vi "BCU参数读取-Auto.vi"(8 "CAN端口":u16(ring), 9 "设备索引号":u16(ring), 10 "CAN卡类型":u32(ring)=21, 11 "Myindex":dbl=1.0) -> (3 "成功":bool)   [LabVIEW 2013] (continued)
                      w1344 = string[][] []
                      w1357 = "总信息" ("section")
                      n843 = local write "路径"(w1343) -> ()
                      n844 = call <vilib>:"Open Config Data.vi"("create file if necessary (T)"=FALSE, "configuration file path"=w1343) -> ("error out"=w1348:errorcluster, "refnum"=w1347:T25)  [unwired: 7 in, 1 out]
                      n845 = call <vilib>:"Get Key Names.vi"("section"=w1357, "error in (no error)"=w1348, "refnum"=w1347) -> ("key names"=w1356:string[], "refnum out"=w1358:T25)  [unwired: 5 in, 2 out]
                      n846 = for {
                        tunnel: w1358 -> [w1364]
                        tunnel: w1357 -> [w1363]
                        tunnel: w1356 -> [w1362] mode=indexing
                        tunnel: [w1361] -> w1353 mode=indexing
                        n847 = call-poly <vilib>:"Read Key.vi"("section"=w1363, "key"=w1362, "refnum"=w1364) -> ("value"=w1361:string)  [unwired: 5 in, 3 out]
                      }
                      n848 = Index Array(array=w1353) -> (element #1=w1346:string, element #2=w1351:string)  [unwired: 2 in]
                      n849 = Decimal String To Number(string=w1346) -> (number=w1345:i32)  [unwired: 2 in, 1 out]
                      n850 = Concatenate Strings("正在读取" ("字符串"), w1351, "的配置文件" ("字符串")) -> (w1349:string)
                      n851 = Build Array(w1349) -> (w1354:string[])
                      n852 = call "表格编辑.vi"("新元素/子数组"=w1354, "活动单元格:单元格背景色"=u32 6618880, "MCListbox引用句柄"=w1360) -> ()  [unwired: 9 out]
                      n853 = local write "项目信息"(w1344) -> ()
                      n854 = local write "项目信息 2"(w1344) -> ()
                    }
                    frame #1 {
                      w1535 = 20 ("长度")
                      w1576 = "主板" ("section")
                      n855 = call <vilib>:"Get Key Names.vi"("section"=w1576, "refnum"=w1575) -> ("key names"=w1377:string[], "refnum out"=w1577:T25)  [unwired: 6 in, 2 out]
                      n856 = for {
                        tunnel: w1577 -> [w1589]
                        tunnel: w1576 -> [w1588]
                        tunnel: w1377 -> [w1587] mode=indexing
                        tunnel: [w1586] -> w1376 mode=indexing
                        n857 = call-poly <vilib>:"Read Key.vi"("section"=w1588, "key"=w1587, "refnum"=w1589) -> ("value"=w1586:string)  [unwired: 5 in, 3 out]
                      }
                      n858 = Search 1D Array(1D array=w1377, element="总电压过高一级" ("元素"), start index (0)=0 ("开始索引(0)")) -> (index of element=w1457:i32)
                      n859 = Search 1D Array(1D array=w1377, element="风机开启温度" ("元素"), start index (0)=w1457) -> (index of element=w1448:i32)
                      n860 = Search 1D Array(1D array=w1377, element="电池串联" ("元素"), start index (0)=w1448) -> (index of element=w1446:i32)
                      n861 = Decrement(x=w1457) -> (x-1=w1574:i32)
                      n862 = Array Subset(array=w1377, index=1 ("索引"), length=w1574) -> (w1422:string[])
                      n863 = Array Subset(array=w1376, index=1 ("索引"), length=w1574) -> (w1419:string[])
                      n864 = Delete From Array(array=w1419, length=7 ("长度"), index=0 ("索引")) -> (deleted portion=w1416:string[], array with subset deleted=w1366:string[])
                      n865 = Delete From Array(array=w1422, length=7 ("长度"), index=0 ("索引")) -> (array with subset deleted=w1375:string[])  [unwired: 1 out]
                      n866 = Search 1D Array(1D array=w1377, element="分流器型号" ("元素")) -> (index of element=w1380:i32)  [unwired: 1 in]
                      n867 = Index Array(array=w1376, index=0 ("索引")) -> (element=w1550:string)
                      n868 = Decimal String To Number(string=w1550) -> (number=w1367:i32)  [unwired: 2 in, 1 out]
                      n869 = Search 1D Array(1D array=w1375, element="主板电池节数" ("元素")) -> (index of element=w1541:i32)  [unwired: 1 in]
                      n870 = Search 1D Array(1D array=w1375, element="主板温度起始值" ("元素")) -> (index of element=w1538:i32)  [unwired: 1 in]
                      n871 = Search 1D Array(1D array=w1375, element="第一个保险通道" ("元素")) -> (index of element=w1537:i32)  [unwired: 1 in]
                      n872 = Search 1D Array(1D array=w1375, element="主板温度个数" ("元素")) -> (index of element=w1539:i32)  [unwired: 1 in]
                      n873 = Search 1D Array(1D array=w1375, element="主板电压起始值" ("元素")) -> (index of element=w1540:i32)  [unwired: 1 in]
                      n874 = Search 1D Array(1D array=w1375, element="第1通道电压个数" ("元素")) -> (index of element=w1536:i32)  [unwired: 1 in]
                      n875 = Index Array(array=w1376, index=w1380) -> (element=w1379:string)
                      n876 = for {
                        N: 4 -> [_]
                        tunnel: w1416 -> [w1585] mode=indexing
                        tunnel: [w1584] -> w1565 mode=indexing
                        n877 = Fract/Exp String To Number(string=w1585) -> (number=w1584:dbl)  [unwired: 3 in, 1 out]
                      }
                      n878 = Increment(x=w1367) -> (x+1=w1549:i32)
                      n879 = Increment(x=w1367) -> (x+1=w1534:i32)
                      n880 = Increment(x=w1367) -> (x+1=w1547:i32)
                      n881 = Increment(x=w1367) -> (x+1=w1548:i32)
                      n882 = global write "读配置文件全局.vi" "从板个数"(w1367) -> ()
                      n883 = local write "从板个数"(w1367) -> ()
                      n884 = Decimal String To Number(string=w1379) -> (number=w1378:i32)  [unwired: 2 in, 1 out]
                      n885 = Index Array(array=w1416, index #1=4 ("索引"), index #2=5 ("索引"), index #3=6 ("索引")) -> (element #1=w1556:string, element #2=w1555:string, element #3=w1554:string)
                      n886 = Index Array(array=w1565) -> (element #1=w1563:dbl, element #2=w1562:dbl, element #3=w1561:dbl, element #4=w1560:dbl)  [unwired: 4 in]
                      n887 = global write "EV05全局变量1.vi" "分流器型号"(w1378) -> ()
                      n888 = Array Subset(array=w1366, index=w1541, length=w1549) -> (w1533:string[])
                      n889 = Array Subset(array=w1366, index=w1540, length=w1548) -> (w1531:string[])
                      n890 = Array Subset(array=w1366, index=w1539, length=w1547) -> (w1530:string[])
                      n891 = Array Subset(array=w1366, index=w1538, length=w1534) -> (w1529:string[])
                      n892 = Array Subset(array=w1366, index=w1537, length=20 ("长度")) -> (w1528:string[])
                      n893 = Array Subset(array=w1366, index=w1536, length=w1535) -> (w1532:string[])
                      n894 = Multiply(x=w1367, y=2) -> (x*y=w1368:i32)
                      n895 = control-ref of="项目信息2"() -> (w1568:refnum<vi>)
                      n896 = Array Subset(array=w1366, index=0 ("索引"), length=w1368) -> (w1365:string[])
                      n897 = Insert Into Array(array=w1533, new element #1=w1532, new element #2=w1531, new element #3=w1530, new element #4=w1529, new element #5=w1528) -> ()  [unwired: 1 in, 1 out]
                      n898 = property class="Clust (严格)"(reference=w1568) -> (reference out=w1566:refnum<vi>, "Value"=w1567:T9)  [unwired: 1 in, 1 out]
                      n899 = Multiply(x=w1367, y=2) -> (x*y=w1372:i32)
                      n900 = Array Subset(array=w1375, index=w1541, length=w1534) -> (w1406:string[])
                      n901 = Array Subset(array=w1375, index=w1540, length=w1534) -> (w1404:string[])
                      n902 = Array Subset(array=w1375, index=w1539, length=w1534) -> (w1403:string[])
                      n903 = Array Subset(array=w1375, index=w1538) -> (w1402:string[])  [unwired: 1 in]
                      n904 = Array Subset(array=w1375, index=w1537, length=w1535) -> (w1401:string[])
                      n905 = Array Subset(array=w1375, index=w1536, length=w1535) -> (w1405:string[])
                      n906 = Array Subset(array=w1375, index=0 ("索引"), length=w1372) -> (w1371:string[])
                      n907 = global write "读配置文件全局.vi" "表格输入"(w1365) -> ()
                      n908 = Build Array(w1371, w1365) -> (w1527:string[][])
                      n909 = Bundle(cluster=w1567, "电池额定容量(A)"=w1563, "使用者"=w1553, "电池实际容量(A)"=w1562, "车架(牌)号"=w1555, "配置文件版本"=w1554, "SOH(%)"=w1560, "SOC(%)"=w1561, "产品编号"=w1556) -> (w1393:T9)  [unwired: 1 in]
                      n910 = Transpose 2D Array(2D array=w1527) -> (transposed array=w1394:string[][])
                      n911 = Multiply(x=w1367, y=4) -> (x*y=w1398:i32)
                      n912 = Insert Into Array(array=w1406, new element #1=w1405, new element #2=w1404, new element #3=w1403, new element #4=w1402, new element #5=w1401) -> (w1400:string[])  [unwired: 1 in]
                      n913 = Add(x=w1398, y=44) -> (x+y=w1396:i32)
                      n914 = local write "项目信息"(w1394) -> ()
                      n915 = property class="Clust (严格)"(reference=w1566, "Value"=w1393) -> ()  [unwired: 1 in, 2 out]
                      n916 = global write "读配置文件全局.vi" "项目信息"(w1393) -> ()
                      n917 = Array Subset(array=w1376, index=w1446, length=15 ("长度")) -> (w1384:string[])
                      n918 = Array Subset(array=w1400, index=0 ("索引"), length=w1396) -> ()  [unwired: 1 out]
                      n919 = Array Subset(array=w1376, index=w1448, length=15 ("长度")) -> (w1453:string[])
                      n920 = Delete From Array(array=w1384, length=4 ("长度"), index=6 ("索引")) -> (deleted portion=w1440:string[], array with subset deleted=w1439:string[])
                      n921 = for {
                        tunnel: w1453 -> [w1581] mode=indexing
                        tunnel: [w1580] -> w1452 mode=indexing
                        n922 = Fract/Exp String To Number(string=w1581) -> (number=w1580:dbl)  [unwired: 3 in, 1 out]
                      }
                      n923 = for {
                        tunnel: w1439 -> [w1579] mode=indexing
                        tunnel: [w1578] -> w1438 mode=indexing
                        n924 = Fract/Exp String To Number(string=w1579) -> (number=w1578:dbl)  [unwired: 3 in, 1 out]
                      }
                      n925 = Array Subset(array=w1376, index=w1457, length=51 ("长度")) -> (w1526:string[])
                      n926 = for {
                        tunnel: w1526 -> [w1583] mode=indexing
                        tunnel: [w1582] -> w1525 mode=indexing
                        n927 = Fract/Exp String To Number(string=w1583) -> (number=w1582:dbl)  [unwired: 3 in, 1 out]
                      }
                      n928 = Index Array(array=w1438) -> (element #1=w1433:dbl, element #2=w1432:dbl, element #3=w1431:dbl, element #4=w1430:dbl, element #5=w1429:dbl, element #6=w1428:dbl, element #7=w1427:dbl, element #8=w1426:dbl, element #9=w1425:dbl, element #10=w1424:dbl, element #11=w1423:dbl)  [unwired: 11 in]
                      n929 = Delete From Array(array=w1452, length=7 ("长度"), index=0 ("索引")) -> (deleted portion=w1389:dbl[], array with subset deleted=w1450:dbl[])
                      n930 = Delete From Array(array=w1525, length=17 ("长度"), index=0 ("索引")) -> (deleted portion=w1386:dbl[], array with subset deleted=w1522:dbl[])
                      n931 = Array To Cluster(array=w1389) -> (cluster=w1451:T26)
                      n932 = global write "读配置文件全局.vi" "加热控制参数"(w1389) -> ()
                      n933 = Index Array(array=w1450) -> (element #1=w1414:dbl, element #2=w1413:dbl, element #3=w1412:dbl, element #4=w1411:dbl, element #5=w1410:dbl, element #6=w1409:dbl, element #7=w1408:dbl, element #8=w1407:dbl)  [unwired: 8 in]
                      n934 = Delete From Array(array=w1522, length=17 ("长度"), index=0 ("索引")) -> (deleted portion=w1385:dbl[], array with subset deleted=w1382:dbl[])
                      n935 = Index Array(array=w1440) -> (element #1=w1437:string, element #2=w1436:string, element #3=w1434:string, element #4=w1435:string)  [unwired: 4 in]
                      n936 = local write "加热控制参数"(w1451) -> ()
                      n937 = global write "读配置文件全局.vi" "一级故障"(w1386) -> ()
                      n938 = local read "一级故障 5"() -> (w1415:T12)
                      n939 = control-ref of="电池信息"() -> (w1444:refnum<vi>)
                      n940 = global write "读配置文件全局.vi" "二级故障"(w1385) -> ()
                      n941 = global write "读配置文件全局.vi" "三级故障"(w1382) -> ()
                      n942 = Bundle(cluster=w1415, "最大允许单体电压"=w1414, "最大允许总电压"=w1410, "最小允许单体电压"=w1413, "最大允许充电电流"=w1412, "最小允许充电电流"=w1411, "最大允许充电温度"=w1409, "最小允许充电温度"=w1408, "电流步长"=w1407) -> (w1388:T12)
                      n943 = property class="Clust (严格)"(reference=w1444) -> (reference out=w1445:refnum<vi>, "Value"=w1443:T13)  [unwired: 1 in, 1 out]
                      n944 = Bundle(cluster=w1443, "电池串联"=w1433, "电池并联"=w1432, "累计放电总安时"=w1426, "电池包额定容量"=w1431, "电池包额定能量(kWh)"=w1430, "电池包额定总电压"=w1429, "累计充电总安时"=w1427, "电池充满次数"=w1424, "电池放空次数"=w1425, "电池充电次数"=w1423, "电池生产日期"=w1434, "电池厂家"=w1437, "电池类型"=w1436, "电池包组号"=w1435, "实际容量"=w1428) -> (w1383:T13)  [unwired: 2 in]
                      n945 = Cluster To Array(cluster=w1388) -> (array=w1387:dbl[])
                      n946 = local write "一级故障 5"(w1388) -> ()
                      n947 = global write "读配置文件全局.vi" "充电控制参数"(w1387) -> ()
                      n948 = Index Array(array=w1386) -> (element #1=w1515:dbl, element #2=w1514:dbl, element #3=w1513:dbl, element #4=w1512:dbl, element #5=w1511:dbl, element #6=w1510:dbl, element #7=w1509:dbl, element #8=w1508:dbl, element #9=w1507:dbl, element #10=w1506:dbl, element #11=w1505:dbl, element #12=w1504:dbl, element #13=w1503:dbl, element #14=w1502:dbl, element #15=w1501:dbl, element #16=w1500:dbl, element #17=w1499:dbl)  [unwired: 17 in]
                      n949 = global write "读配置文件全局.vi" "电池信息"(w1383) -> ()
                      n950 = Index Array(array=w1385) -> (element #1=w1482:dbl, element #2=w1483:dbl, element #3=w1484:dbl, element #4=w1485:dbl, element #5=w1486:dbl, element #6=w1487:dbl, element #7=w1488:dbl, element #8=w1489:dbl, element #9=w1490:dbl, element #10=w1491:dbl, element #11=w1492:dbl, element #12=w1493:dbl, element #13=w1494:dbl, element #14=w1495:dbl, element #15=w1496:dbl, element #16=w1497:dbl, element #17=w1498:dbl)  [unwired: 17 in]
                      n951 = Index Array(array=w1382) -> (element #1=w1477:dbl, element #2=w1476:dbl, element #3=w1475:dbl, element #4=w1474:dbl, element #5=w1473:dbl, element #6=w1472:dbl, element #7=w1471:dbl, element #8=w1470:dbl, element #9=w1469:dbl, element #10=w1468:dbl, element #11=w1467:dbl, element #12=w1466:dbl, element #13=w1465:dbl, element #14=w1464:dbl, element #15=w1463:dbl, element #16=w1462:dbl, element #17=w1461:dbl)  [unwired: 17 in]
                      n952 = control-ref of="一级故障 3"() -> (w1460:refnum<vi>)
                      n953 = control-ref of="一级故障 2"() -> (w1479:refnum<vi>)
                      n954 = property class="Clust (严格)"(reference=w1479) -> (reference out=w1481:refnum<vi>, "Value"=w1480:T10)  [unwired: 1 in, 1 out]
                      n955 = property class="Clust (严格)"(reference=w1460) -> (reference out=w1459:refnum<vi>, "Value"=w1478:T10)  [unwired: 1 in, 1 out]
                      n956 = property class="Clust (严格)"(reference=w1445, "Value"=w1383) -> ()  [unwired: 1 in, 2 out]
                      n957 = Bundle(cluster=w1480, "总电压过高"=w1482, "整组电压不均衡"=w1486, "SOC过高"=w1494, "单体电压过高"=w1490, "总电压过低"=w1483, "温度过高"=w1484, "温度过低"=w1485, "单组电压不均衡"=w1487, "整组温度不均衡"=w1488, "单组温度不均衡"=w1489, "单体电压过低"=w1491, "充电电流过高"=w1492, "放电电流过高"=w1493, "SOC过低"=w1495, "内阻过大"=w1496, "极柱温度过高"=w1497, "SOH过低"=w1498) -> (w1391:T10)
                      n958 = property class="Clust (严格)"(reference=w1481, "Value"=w1391) -> ()  [unwired: 1 in, 2 out]
                      n959 = Bundle(cluster=w1478, "总电压过高"=w1477, "整组电压不均衡"=w1473, "SOC过高"=w1465, "单体电压过高"=w1469, "总电压过低"=w1476, "温度过高"=w1475, "温度过低"=w1474, "单组电压不均衡"=w1472, "整组温度不均衡"=w1471, "单组温度不均衡"=w1470, "单体电压过低"=w1468, "充电电流过高"=w1467, "放电电流过高"=w1466, "SOC过低"=w1464, "内阻过大"=w1463, "极柱温度过高"=w1462, "SOH过低"=w1461) -> (w1390:T10)
                      n960 = property class="Clust (严格)"(reference=w1459, "Value"=w1390) -> ()  [unwired: 1 in, 2 out]
                      n961 = control-ref of="一级故障"() -> (w1518:refnum<vi>)
                      n962 = property class="Clust (严格)"(reference=w1518) -> (reference out=w1516:refnum<vi>, "Value"=w1517:T10)  [unwired: 1 in, 1 out]
                      n963 = Bundle(cluster=w1517, "总电压过高"=w1515, "整组电压不均衡"=w1511, "SOC过高"=w1503, "单体电压过高"=w1507, "总电压过低"=w1514, "温度过高"=w1513, "温度过低"=w1512, "单组电压不均衡"=w1510, "整组温度不均衡"=w1509, "单组温度不均衡"=w1508, "单体电压过低"=w1506, "充电电流过高"=w1505, "放电电流过高"=w1504, "SOC过低"=w1502, "内阻过大"=w1501, "极柱温度过高"=w1500, "SOH过低"=w1499) -> (w1392:T10)
                      n964 = property class="Clust (严格)"(reference=w1516, "Value"=w1392) -> ()  [unwired: 1 in, 2 out]
                    }
                    frame #2 {
                      w1654 = 1 ("索引")
                      # "均衡计算-电压高阀值1级"
                      n965 = call <vilib>:"Get Section Names.vi"("refnum"=w1669) -> ("section names"=w1670:string[], "refnum out"=w1674:T25)  [unwired: 8 in, 1 out]
                      n966 = local read "从板号"() -> (w1652:u8)
                      n967 = Delete From Array(array=w1670, length=2 ("长度"), index=0 ("索引")) -> (array with subset deleted=w1673:string[])  [unwired: 1 out]
                      n968 = for {
                        tunnel: w1673 -> [w1690] mode=indexing
                        tunnel: w1674 -> [w1691]
                        tunnel: [w1683] -> w1651 mode=indexing
                        tunnel: [w1682] -> w1595
                        n969 = call <vilib>:"Get Key Names.vi"("section"=w1690, "refnum"=w1691) -> ("key names"=w1682:string[], "refnum out"=w1689:T25)  [unwired: 6 in, 2 out]
                        n970 = for {
                          tunnel: w1682 -> [w1695] mode=indexing
                          tunnel: w1690 -> [w1694]
                          tunnel: w1689 -> [w1693]
                          tunnel: [w1692] -> w1683 mode=indexing
                          n971 = call-poly <vilib>:"Read Key.vi"("section"=w1694, "key"=w1695, "refnum"=w1693) -> ("value"=w1692:string)  [unwired: 5 in, 3 out]
                        }
                        n972 = Index Array(array=w1683, index=0 ("索引")) -> (element=w1686:string)
                        n973 = local read "输出数组"() -> (w1687:string[][])
                        n974 = Decimal String To Number(string=w1686) -> (number=w1685:i32)  [unwired: 2 in, 1 out]
                        n975 = Decrement(x=w1685) -> (x-1=w1681:i32)
                        n976 = Replace Array Subset(array=w1687, new element=w1683, index (col)=w1681) -> (w1684:string[][])  [unwired: 1 in]
                        n977 = local write "输出数组"(w1684) -> ()
                      }
                      "key names" <- w1595
                      n978 = Decrement(x=w1652) -> (x-1=w1668:u8)
                      n979 = Index Array(array=w1651, index (row)=w1668) -> (element=w1594:string[])  [unwired: 1 in]
                      n980 = Search 1D Array(1D array=w1595, element="风机开启温度" ("元素")) -> (index of element=w1657:i32)  [unwired: 1 in]
                      n981 = Search 1D Array(1D array=w1595, element="电压过高一级" ("元素"), start index (0)=w1657) -> (index of element=w1620:i32)
                      n982 = Search 1D Array(1D array=w1595, element="均衡计算-电压高阀值1级" ("元素"), start index (0)=w1620) -> (index of element=w1618:i32)
                      n983 = Array Subset(array=w1594, index=w1618, length=17 ("长度")) -> (w1617:string[])
                      n984 = Decrement(x=w1657) -> (x-1=w1655:i32)
                      n985 = Array Subset(array=w1594, index=w1654, length=w1655) -> (w1592:string[])
                      n986 = Array Subset(array=w1594, index=w1620, length=21 ("长度")) -> (w1666:string[])
                      n987 = Array Subset(array=w1595, index=w1654, length=w1655) -> (w1631:string[])
                      n988 = Index Array(array=w1594, index=0 ("索引")) -> (element=w1626:string)
                      n989 = Array Subset(array=w1594, index=w1657, length=7 ("长度")) -> (w1660:string[])
                      n990 = for {
                        tunnel: w1617 -> [w1676] mode=indexing
                        tunnel: [w1675] -> w1616 mode=indexing
                        n991 = Fract/Exp String To Number(string=w1676) -> (number=w1675:dbl)  [unwired: 3 in, 1 out]
                      }
                      n992 = for {
                        tunnel: w1666 -> [w1678] mode=indexing
                        tunnel: [w1677] -> w1667 mode=indexing
                        n993 = Fract/Exp String To Number(string=w1678) -> (number=w1677:dbl)  [unwired: 3 in, 1 out]
                      }
                      n994 = Decimal String To Number(string=w1626) -> (number=w1625:i32)  [unwired: 2 in, 1 out]
                      n995 = for {
                        tunnel: w1660 -> [w1680] mode=indexing
                        tunnel: [w1679] -> w1628 mode=indexing
                        n996 = Fract/Exp String To Number(string=w1680) -> (number=w1679:dbl)  [unwired: 3 in, 1 out]
                      }
                      n997 = global write "读配置文件全局2.vi" "从板板号"(w1625) -> ()
                      n998 = Delete From Array(array=w1667, length=7 ("长度"), index=0 ("索引")) -> (deleted portion=w1630:dbl[], array with subset deleted=w1663:dbl[])
                      n999 = Array To Cluster(array=w1628) -> (cluster=w1650:T26)
                      n1000 = global write "读配置文件全局2.vi" "加热控制参数"(w1628) -> ()
                      n1001 = Delete From Array(array=w1663, length=7 ("长度"), index=0 ("索引")) -> (deleted portion=w1623:dbl[], array with subset deleted=w1624:dbl[])
                      n1002 = local write "加热控制参数"(w1650) -> ()
                      n1003 = Array To Cluster(array=w1630) -> (cluster=w1634:T26)
                      n1004 = Array To Cluster(array=w1624) -> (cluster=w1632:T26)
                      n1005 = Array To Cluster(array=w1623) -> (cluster=w1633:T26)
                      n1006 = global write "读配置文件全局2.vi" "三级故障阀值"(w1624) -> ()
                      n1007 = global write "读配置文件全局2.vi" "一级故障阀值"(w1630) -> ()
                      n1008 = global write "读配置文件全局2.vi" "二级故障阀值"(w1623) -> ()
                      n1009 = local write "一级故障 6"(w1634) -> ()
                      n1010 = local write "一级故障 8"(w1632) -> ()
                      n1011 = local write "一级故障 7"(w1633) -> ()
                      n1012 = Search 1D Array(1D array=w1631, element="第1通道电压个数" ("元素")) -> (index of element=w1642:i32)  [unwired: 1 in]
                      n1013 = Search 1D Array(1D array=w1631, element="电压个数" ("元素")) -> ()  [unwired: 1 in, 1 out]
                      n1014 = Search 1D Array(1D array=w1631, element="温度个数" ("元素")) -> (index of element=w1644:i32)  [unwired: 1 in]
                      n1015 = Search 1D Array(1D array=w1631, element="第一个保险通道" ("元素")) -> (index of element=w1643:i32)  [unwired: 1 in]
                      n1016 = Array Subset(array=w1592, length=2 ("长度")) -> (w1639:string[])  [unwired: 1 in]
                      n1017 = Array Subset(array=w1592, index=w1644, length=2 ("长度")) -> (w1637:string[])
                      n1018 = Array Subset(array=w1592, index=w1643, length=20 ("长度")) -> (w1636:string[])
                      n1019 = Array Subset(array=w1592, index=w1642, length=20 ("长度")) -> (w1638:string[])
                      n1020 = Array Subset(array=w1592, length=27 ("长度")) -> (w1591:string[])  [unwired: 1 in]
                      n1021 = Insert Into Array(array=w1639, new element #1=w1638, new element #2=w1637, new element #3=w1636) -> ()  [unwired: 1 in, 1 out]
                      n1022 = Build Array(string[] ["电压个数", "温度个数", "第一个保险通道", "第一个保险位置", "第二个保险通道", "第二个保险位置", "第三个保险通道", "第三个保险位置", "第四个保险通道", "第四个保险位置", "第五个保险通道", "第五个保险位置", "第六个保险通道", "第六个保险位置", "第七个保险通道", "第七个保险位置", "第八个保险通道", "第八个保险位置", "第九个保险通道", "第九个保险位置", "第十个保险通道", "第十个保险位置", "第1通道电压个数", "第2通道电压个数", "第3通道电压个数", "第4通道电压个数", "第5通道电压个数"], w1591) -> (w1635:string[][])
                      n1023 = global write "读配置文件全局2.vi" "表格"(w1591) -> ()
                      n1024 = Index Array(array=w1616) -> (element #1=w1613:dbl, element #2=w1612:dbl, element #3=w1611:dbl, element #4=w1610:dbl, element #5=w1609:dbl, element #6=w1608:dbl, element #7=w1607:dbl, element #8=w1606:dbl, element #9=w1605:dbl, element #10=w1604:dbl, element #11=w1603:dbl, element #12=w1602:dbl, element #13=w1601:dbl, element #14=w1600:dbl, element #15=w1599:dbl, element #16=w1598:dbl, element #17=w1597:dbl, element #18=w1596:dbl)  [unwired: 18 in]
                      n1025 = Transpose 2D Array(2D array=w1635) -> (transposed array=w1629:string[][])
                      n1026 = local write "项目信息 2"(w1629) -> ()
                      n1027 = local read "均衡参数"() -> (w1615:T17)
                      n1028 = Bundle(cluster=w1615, "充电结束电压(90%)"=w1606, "充电结束电压(91%)"=w1605, "充电结束电压(92%)"=w1604, "充电结束电压(93%)"=w1603, "充电结束电压(94%)"=w1602, "均衡计算-电压高阀值1级"=w1613, "均衡计算-电压高阀值2级"=w1612, "均衡计算-电压低阀值1级"=w1611, "均衡计算-电压低阀值2级"=w1610, "均衡计算-最低电压阀值"=w1609, "均衡停止-最低电压阀值"=w1608, "均衡计算-电压极差阀值"=w1607, "充电结束电压(95%)"=w1601, "充电结束电压(96%)"=w1600, "充电结束电压(97%)"=w1599, "充电结束电压(98%)"=w1598, "充电结束电压(99%)"=w1597, "充电结束电压(100%)"=w1596) -> (w1614:T17)
                      n1029 = local write "均衡参数"(w1614) -> ()
                    }
                    frame #3 {
                      n1030 = call <vilib>:"Unset Busy.vi"() -> ()  [unwired: 11 in, 1 out]
                      n1031 = Build Array("读取完成") -> (w1699:string[])
                      n1032 = property on="全部写入" class="Bool (严格)"("DisabledEnum"=0) -> ()  [unwired: 2 in, 2 out]
                      n1033 = call "表格编辑.vi"("新元素/子数组"=w1699, "活动单元格:单元格背景色"=u32 6618880, "MCListbox引用句柄"=w1696) -> ()  [unwired: 9 out]
                    }
                  }
                }
              }
            }
            frame #2 {
              (unwired) "均衡参数"
              # "去掉加热控制信息 20140106"
              n1034 = local read "主从选择"() -> (w1704:enum32{"主板", "从板"})
              n1035 = case shown="\"主板\", 默认" w1704 {
                tunnel: [string[] ["项目信息", "一级故障阀值", "二级故障阀值", "三级故障阀值", "加热控制信息", "充电控制信息", "电池信息", "二维码"] string[] ["从板信息", "一级故障阀值", "二级故障阀值", "三级故障阀值", "二维码"]] -> w1703
                frame "主板", Default {
                }
                frame "从板" {
                }
              }
              n1036 = Array Size(array=w1703) -> (size(s)=w1702:i32)
              n1037 = for {
                tunnel: w1703 -> [w1720] mode=indexing
                tunnel: w1704 -> [w1708]
                tunnel: w1702 -> [w1712]
                tunnel: [w1707] -> w1701
                i -> [w1709]
                n1038 = case shown="\"主板\", 默认" w1708 {
                  tunnel: [w2017 w2048] -> w1714
                  tunnel: [w2016 w2049] -> w1715
                  tunnel: w1720 -> [w2013 w2045]
                  tunnel: [u8 0 ("板号") w2046] -> w1719
                  tunnel: [u8 0 ("板号") u8 0 ("板号")] -> w1718
                  tunnel: [w2012 w2044] -> w1716
                  frame "主板", Default {
                    n1039 = case shown="\"项目信息\"" w2013 {
                      tunnel: [_ u8[] [1, 2, 3, 4, 5, 6, 13, 8, 7, 9, 10, 11, 12] u8[] [1] u8[] [1] u8[] [2] u8[] [3] u8[] [1] u8[] [2] u8[] [1, 2, 3] u8[] [1, 2, 3, 4]] -> w2017
                      tunnel: [_ u8 128 ("命令") u8 140 ("命令") u8 129 ("命令") u8 129 ("命令") u8 129 ("命令") u8 130 ("命令") u8 130 ("命令") u8 131 ("命令") u8 132 ("命令")] -> w2016
                      tunnel: [_ string[] ["产品编号", "电压个数", "通道电压数", "电压起始值", "温度个数", "温度起始值", "保险位置", "电池额定实际容量", "SOC", "配置文件版本", "参数修改记录", "车牌号", "SOH"] string[] ["读二维码"] string[] ["一级故障阀值"] string[] ["二级故障阀值"] string[] ["三级故障阀值"] string[] ["加热控制参数"] string[] ["充电控制参数"] _ string[] ["电池信息1", "电池包组号", "充放电安时", "电池充放电次数"]] -> w2012
                      frame "假", Default {
                      }
                      frame "项目信息" {
                      }
                      frame "二维码" {
                      }
                      frame "一级故障阀值" {
                      }
                      frame "二级故障阀值" {
                      }
                      frame "三级故障阀值" {
                      }
                      frame "加热控制信息" {
                      }
                      frame "充电控制信息" {
                      }
                      frame "历史信息" {
                      }
                      frame "电池信息" {
                      }
                    }
                  }
                  frame "从板" {
                    n1040 = case shown="\"二维码\"" w2045 {
                      tunnel: [_ u8 0 ("命令") u8 10 ("命令") u8 2 ("命令") u8 2 ("命令") u8 2 ("命令") u8 3 ("命令") u8 6 ("命令")] -> w2049
                      tunnel: [_ u8[] [6, 1, 2, 3, 4, 5] u8[] [1] u8[] [1] u8[] [2] u8[] [3] u8[] [1, 2, 3, 4, 5, 6, 7] u8[] [1, 2]] -> w2048
                      tunnel: [_ string[] ["从板号", "电压起始值", "通道电压节数", "保险位置", "温度起始值", "加热控制参数"] string[] ["读二维码"] string[] ["一级故障阀值"] string[] ["二级故障阀值"] string[] ["三级故障阀值"] string[] ["电池包信息1", "电池包序号", "充放电安时", "充电次数时间", "SOC", "车牌号", "充电参数"] string[] ["均衡阀值", "充电结束电压"]] -> w2044
                      frame "假", Default {
                      }
                      frame "从板信息" {
                      }
                      frame "二维码" {
                      }
                      frame "一级故障阀值" {
                      }
                      frame "二级故障阀值" {
                      }
                      frame "三级故障阀值" {
                      }
                      frame "快换参数" {
                      }
                      frame "均衡参数" {
                      }
                    }
                    n1041 = local read "从板号"() -> (w2046:u8)
                  }
                }
                n1042 = Increment(x=w1709) -> (x+1=w1711:i32)
                n1043 = Equal?(x=w1712, y=w1711) -> (x = y?=w1710:bool)
                n1044 = case shown="\"从板\"" w1708 {
                  tunnel: w1709 -> [w1983 w1997]
                  frame "主板", Default {
                    n1045 = case shown="0, 默认" w1983 {
                      tunnel: [T8."项目信息" ("主从板") T8."一级故障阀值" ("主从板") T8."二级故障阀值" ("主从板") T8."三级故障阀值" ("主从板") T8."控制参数" ("主从板") T8."电池信息" ("主从板")] -> w1982
                      frame 0, Default {
                        n1046 = local write "1"(TRUE ("1")) -> ()
                      }
                      frame 1 {
                        n1047 = local write "1 2"(TRUE ("1 2")) -> ()
                      }
                      frame 2 {
                        n1048 = local write "1 3"(TRUE ("1 3")) -> ()
                      }
                      frame 3 {
                        n1049 = local write "1 4"(TRUE ("1 4")) -> ()
                      }
                      frame 4, 5 {
                        n1050 = local write "1 5"(TRUE ("1 5")) -> ()
                      }
                      frame 6 {
                        n1051 = local write "1 11"(TRUE ("1 11")) -> ()
                      }
                    }
                    n1052 = local write "主板2"(w1982) -> ()
                  }
                  frame "从板" {
                    n1053 = case shown="4" w1997 {
                      tunnel: [T19."从板信息" ("等级 2") T19."从板信息" ("等级 2") T19."一级故障阀值" ("等级 2") T19."二级故障阀值" ("等级 2") T19."三级故障阀值" ("等级 2") T19."快换参数" ("等级 2") T14."从板信息" ("等级 2")] -> w1996
                      frame 99, Default {
                        n1054 = local write "1 6"(TRUE ("1 6")) -> ()
                      }
                      frame 0 {
                        n1055 = local write "1 6"(TRUE ("1 6")) -> ()
                      }
                      frame 1 {
                        n1056 = local write "1 7"(TRUE ("1 7")) -> ()
                      }
                      frame 2 {
                        n1057 = local write "1 8"(TRUE ("1 8")) -> ()
                      }
                      frame 3 {
                        n1058 = local write "1 9"(TRUE ("1 9")) -> ()
                      }
                      frame 5 {
                        n1059 = local write "1 10"(TRUE ("1 10")) -> ()
                      }
                      frame 4 {
                        n1060 = local write "1 12"(TRUE ("1 10")) -> ()
                      }
                    }
                    n1061 = local write "等级 2"(w1996) -> ()
                  }
                }
                n1062 = Array Size(array=w1714) -> (size(s)=w1713:i32)
                n1063 = local write "命令"(w1715) -> ()
                n1064 = Build Array(w1718) -> (w1717:u8[])
                n1065 = while {
                  tunnel: w1715 -> [w1752]
                  tunnel: w1719 -> [w1751]
                  tunnel: w1717 -> [w1750]
                  tunnel: w1713 -> [w1746]
                  tunnel: w1710 -> [w1749]
                  tunnel: w1708 -> [w1743]
                  tunnel: [w1742] -> w1707
                  shift-right: [w1741] -> _
                  shift-left: w1716 -> [w1722]
                  shift-right: [w1732] -> _
                  shift-left: w1714 -> [w1721]
                  i -> [w1747]
                  stop <- w1742 stop-if-true
                  n1066 = local read "强制终止读写标记"() -> (w1738:bool)
                  n1067 = Array Size(array=w1722) -> (size(s)=w1740:i32)
                  n1068 = Increment(x=w1747) -> (x+1=w1748:i32)
                  n1069 = Greater Than 0?(x=w1740) -> (x > 0?=w1739:bool)
                  n1070 = Equal?(x=w1746, y=w1748) -> (x = y?=w1744:bool)
                  n1071 = Not(x=w1738) -> (.not. x?=w1737:bool)
                  n1072 = And(x=w1737, y=w1739) -> (x .and. y?=w1736:bool)
                  n1073 = Delete From Array(array=w1722, length=1 ("长度"), index=0 ("索引")) -> (deleted portion=w1728:string[], array with subset deleted=w1733:string[])
                  n1074 = Index Array(array=w1728, index=0 ("索引")) -> (element=w1726:string)
                  n1075 = Delete From Array(array=w1721, length=1 ("长度"), index=0 ("索引")) -> (deleted portion=w1724:u8[], array with subset deleted=w1729:u8[])
                  n1076 = Index Array(array=w1724, index=0 ("索引")) -> (element=w1723:u8)
                  n1077 = case shown="真" w1736 {
                    tunnel: w1752 -> [_ w1768]
                    tunnel: w1723 -> [_ w1767]
                    tunnel: w1751 -> [_ w1766]
                    tunnel: w1750 -> [_ w1765]
                    tunnel: w1726 -> [_ w1764]
                    tunnel: w1749 -> [_ w1763]
                    tunnel: w1744 -> [_ w1762]
                    tunnel: w1743 -> [_ w1761]
                    tunnel: [string[] [] w1757] -> w1741
                    tunnel: w1733 -> [_ w1760]
                    tunnel: [u8[] [] w1755] -> w1732
                    tunnel: w1729 -> [_ w1759]
                    tunnel: w1722 -> [_ w1758]
                    tunnel: w1721 -> [_ w1756]
                    frame False {
                    }
                    frame True {
                      n1078 = while {
                        tunnel: w1768 -> [w1784]
                        tunnel: w1767 -> [w1783]
                        tunnel: w1766 -> [w1782]
                        tunnel: w1765 -> [w1781]
                        tunnel: w1764 -> [w1779]
                        tunnel: w1763 -> [w1778]
                        tunnel: w1762 -> [w1777]
                        tunnel: w1761 -> [w1776]
                        tunnel: w1760 -> [w1772]
                        tunnel: w1759 -> [w1770]
                        tunnel: w1758 -> [w1773]
                        tunnel: [w1774] -> w1757
                        tunnel: w1756 -> [w1771]
                        tunnel: [w1769] -> w1755
                        i -> [w1775]
                        stop <- w1780 stop-if-true
                        n1079 = stacked-sequence {
                          seq-local: [_ _ _ _ w1932 _ _] -> [_ _ _ _ _ w1948 _]
                          tunnel: w1784 -> [_ _ _ w1923 _ _ _]
                          tunnel: w1783 -> [_ _ _ w1922 _ _ _]
                          tunnel: w1782 -> [_ _ _ w1921 _ _ _]
                          tunnel: w1781 -> [_ _ _ w1920 _ _ _]
                          tunnel: [_ _ _ _ w1933 _ _] -> w1780
                          tunnel: w1779 -> [w1786 _ _ _ _ w1947 _]
                          tunnel: w1778 -> [_ _ _ _ _ _ w1975]
                          tunnel: w1777 -> [_ _ _ _ _ _ w1973]
                          tunnel: w1776 -> [w1785 _ _ _ _ _ _]
                          tunnel: w1775 -> [_ _ _ _ _ _ _]
                          tunnel: [_ _ _ _ _ w1946 _] -> w1774
                          tunnel: w1773 -> [_ _ _ _ _ w1945 _]
                          tunnel: w1772 -> [_ _ _ _ _ w1944 _]
                          tunnel: w1771 -> [_ _ _ _ _ w1943 _]
                          tunnel: w1770 -> [_ _ _ _ _ w1942 _]
                          tunnel: [_ _ _ _ _ w1941 _] -> w1769
                          frame #0 {
                            n1080 = case shown="\"从板\"" w1785 {
                              tunnel: w1786 -> [w1787 w1878]
                              frame "主板", Default {
                                n1081 = case shown="\"电压个数\"" w1787 {
                                frame "假", Default {
                                }
                                frame "产品编号" {
                                n1082 = control-ref of="产品编号"() -> (w1789:refnum<vi>)
                                n1083 = property class="Str"(reference=w1789, "Value"="") -> ()  [unwired: 1 in, 2 out]
                                }
                                frame "电压个数" {
                                n1084 = local read "从板个数"() -> (w1790:dbl)
                                n1085 = control-ref of="项目信息"() -> (w1794:refnum<vi>)
                                n1086 = for {
                                N: w1790 -> [_]
                                tunnel: [""] -> w1793 mode=indexing
                                }
                                n1087 = call "表格数据输入-8.6.vi"("行数"=u32 0, "列数"=u32 1, "字符串数组"=w1793, "表格引用"=w1794) -> ()  [unwired: 8 in]
                                }
                                frame "通道电压数" {
                                n1088 = disable-structure shown="禁用" {
                                frame Disabled {
                                n1089 = control-ref of="项目信息"() -> (w1800:refnum<vi>)
                                n1090 = for {
                                N: 20 -> [_]
                                tunnel: [""] -> w1799 mode=indexing
                                }
                                n1091 = local read "从板个数"() -> (w1801:dbl)
                                n1092 = Increment(x=w1801) -> (x+1=w1797:dbl)
                                n1093 = call "表格数据输入-8.6.vi"("行数"=w1797, "列数"=u32 1, "字符串数组"=w1799, "表格引用"=w1800) -> ()  [unwired: 8 in]
                                }
                                frame Enabled {
                                }
                                }
                                }
                                frame "电压起始值" {
                                n1094 = disable-structure shown="禁用" {
                                frame Disabled {
                                n1095 = local read "从板个数"() -> (w1805:dbl)
                                n1096 = Increment(x=w1805) -> (x+1=w1804:dbl)
                                n1097 = control-ref of="项目信息"() -> (w1811:refnum<vi>)
                                n1098 = for {
                                N: w1804 -> [_]
                                tunnel: [""] -> w1810 mode=indexing
                                }
                                n1099 = Multiply(x=u8 1, y=w1805) -> (x*y=w1807:dbl)
                                n1100 = Add(x=w1807, y=u8 21) -> (x+y=w1803:dbl)
                                n1101 = call "表格数据输入-8.6.vi"("行数"=w1803, "列数"=u32 1, "字符串数组"=w1810, "表格引用"=w1811) -> ()  [unwired: 8 in]
                                }
                                frame Enabled {
                                }
                                }
                                }
                                frame "温度个数" {
                                n1102 = local read "从板个数"() -> (w1815:dbl)
                                n1103 = Increment(x=w1815) -> (x+1=w1814:dbl)
                                n1104 = control-ref of="项目信息"() -> (w1821:refnum<vi>)
                                n1105 = for {
                                N: w1814 -> [_]
                                tunnel: [""] -> w1820 mode=indexing
                                }
                                n1106 = Multiply(x=u8 2, y=w1815) -> (x*y=w1817:dbl)
                                n1107 = Add(x=w1817, y=u8 22) -> (x+y=w1813:dbl)
                                n1108 = call "表格数据输入-8.6.vi"("行数"=w1813, "列数"=u32 1, "字符串数组"=w1820, "表格引用"=w1821) -> ()  [unwired: 8 in]
                                }
                                frame "温度起始值" {
                                n1109 = disable-structure shown="禁用" {
                                frame Disabled {
                                n1110 = local read "从板个数"() -> (w1825:dbl)
                                n1111 = Increment(x=w1825) -> (x+1=w1824:dbl)
                                n1112 = control-ref of="项目信息"() -> (w1831:refnum<vi>)
                                n1113 = for {
                                N: w1824 -> [_]
                                tunnel: [""] -> w1830 mode=indexing
                                }
                                n1114 = Multiply(x=u8 3, y=w1825) -> (x*y=w1827:dbl)
                                n1115 = Add(x=w1827, y=u8 23) -> (x+y=w1823:dbl)
                                n1116 = call "表格数据输入-8.6.vi"("行数"=w1823, "列数"=u32 1, "字符串数组"=w1830, "表格引用"=w1831) -> ()  [unwired: 8 in]
                                }
                                frame Enabled {
                                }
                                }
                                }
                                frame "保险位置" {
                                n1117 = local read "从板个数"() -> (w1835:dbl)
                                n1118 = control-ref of="项目信息"() -> (w1841:refnum<vi>)
                                n1119 = for {
                                N: 10 -> [_]
                                tunnel: [""] -> w1840 mode=indexing
                                }
                                n1120 = Multiply(x=u8 4, y=w1835) -> (x*y=w1837:dbl)
                                n1121 = Add(x=w1837, y=u8 24) -> (x+y=w1834:dbl)
                                n1122 = call "表格数据输入-8.6.vi"("行数"=w1834, "列数"=u32 1, "字符串数组"=w1840, "表格引用"=w1841) -> ()  [unwired: 8 in]
                                }
                                frame "电池额定实际容量" {
                                w1843 = 0.0 ("值")
                                n1123 = control-ref of="电池实际容量(A)"() -> (w1844:refnum<vi>)
                                n1124 = control-ref of="电池额定容量(A)"() -> (w1845:refnum<vi>)
                                n1125 = property class="DigNum (严格)"(reference=w1844, "Value"=w1843) -> ()  [unwired: 1 in, 2 out]
                                n1126 = property class="DigNum (严格)"(reference=w1845, "Value"=w1843) -> ()  [unwired: 1 in, 2 out]
                                }
                                frame "SOC" {
                                n1127 = control-ref of="SOC(%)"() -> (w1846:refnum<vi>)
                                n1128 = property class="DigNum (严格)"(reference=w1846, "Value"=0.0 ("值")) -> ()  [unwired: 1 in, 2 out]
                                }
                                frame "配置文件版本" {
                                n1129 = control-ref of="配置文件版本"() -> (w1848:refnum<vi>)
                                n1130 = property class="Str"(reference=w1848, "Value"="" ("值")) -> ()  [unwired: 1 in, 2 out]
                                }
                                frame "参数修改记录" {
                                n1131 = control-ref of="使用者"() -> (w1851:refnum<vi>)
                                n1132 = control-ref of="系统时钟"() -> (w1852:refnum<vi>)
                                n1133 = property class="DigNum (严格)"(reference=w1851, "Value"=0.0 ("值")) -> ()  [unwired: 1 in, 2 out]
                                n1134 = property class="Str"(reference=w1852, "Value"="" ("值")) -> ()  [unwired: 1 in, 2 out]
                                }
                                frame "校正时钟" {
                                n1135 = control-ref of="系统时钟"() -> (w1854:refnum<vi>)
                                n1136 = property class="Str"(reference=w1854, "Value"="" ("值")) -> ()  [unwired: 1 in, 2 out]
                                }
                                frame "车牌号" {
                                n1137 = control-ref of="车架(牌)号"() -> (w1856:refnum<vi>)
                                n1138 = property class="Str"(reference=w1856, "Value"="" ("值")) -> ()  [unwired: 1 in, 2 out]
                                }
                                frame "SOH" {
                                n1139 = control-ref of="SOH(%)"() -> (w1859:refnum<vi>)
                                n1140 = property class="DigNum (严格)"(reference=w1859, "Value"=0.0 ("值")) -> ()  [unwired: 1 in, 2 out]
                                }
                                frame "一级故障阀值" {
                                n1141 = local write "一级故障"(T10 {"总电压过高"=0.0, "整组电压不均衡"=0.0, "SOC过高"=0.0, "单体电压过高"=0.0, "总电压过低"=0.0, "温度过高"=0.0, "温度过低"=0.0, "单组电压不均衡"=0.0, "整组温度不均衡"=0.0, "单组温度不均衡"=0.0, "单体电压过低"=0.0, "充电电流过高"=0.0, "放电电流过高"=0.0, "SOC过低"=0.0, "内阻过大"=0.0, "极柱温度过高"=0.0, "SOH过低"=0.0} ("一级故障")) -> ()
                                }
                                frame "二级故障阀值" {
                                n1142 = local write "一级故障 2"(T10 {"总电压过高"=0.0, "整组电压不均衡"=0.0, "SOC过高"=0.0, "单体电压过高"=0.0, "总电压过低"=0.0, "温度过高"=0.0, "温度过低"=0.0, "单组电压不均衡"=0.0, "整组温度不均衡"=0.0, "单组温度不均衡"=0.0, "单体电压过低"=0.0, "充电电流过高"=0.0, "放电电流过高"=0.0, "SOC过低"=0.0, "内阻过大"=0.0, "极柱温度过高"=0.0, "SOH过低"=0.0} ("一级故障")) -> ()
                                }
                                frame "三级故障阀值" {
                                n1143 = local write "一级故障 3"(T10 {"总电压过高"=0.0, "整组电压不均衡"=0.0, "SOC过高"=0.0, "单体电压过高"=0.0, "总电压过低"=0.0, "温度过高"=0.0, "温度过低"=0.0, "单组电压不均衡"=0.0, "整组温度不均衡"=0.0, "单组温度不均衡"=0.0, "单体电压过低"=0.0, "充电电流过高"=0.0, "放电电流过高"=0.0, "SOC过低"=0.0, "内阻过大"=0.0, "极柱温度过高"=0.0, "SOH过低"=0.0} ("一级故障")) -> ()
                                }
                                frame "加热控制参数" {
                                n1144 = local write "加热控制参数"(T11 {"风机开启温度"=0.0, "风机关闭温度"=0.0, "加热开启温度"=0.0, "加热关闭温度"=0.0, "风机开启温差"=0.0, "风机关闭温差"=0.0, "加热关闭温差"=0.0} ("加热控制参数")) -> ()
                                }
                                frame "充电控制参数" {
                                n1145 = local write "一级故障 5"(T12 {"最大允许单体电压"=0.0, "最大允许总电压"=0.0, "最小允许单体电压"=0.0, "最大允许充电电流"=0.0, "最小允许充电电流"=0.0, "最大允许充电温度"=0.0, "最小允许充电温度"=0.0, "电流步长"=0.0} ("一级故障 5")) -> ()
                                }
                                frame "电池信息1" {
                                w1865 = ""
                                w1866 = 0.0 ("电池串联")
                                n1146 = local read "电池信息"() -> (w1868:T13)
                                n1147 = Bundle By Name(cluster=w1868, "电池串联"=w1866, "电池并联"=w1866, "电池包额定容量"=w1866, "电池包额定能量(kWh)"=w1866, "电池包额定总电压"=w1866, "实际容量"=w1866, "电池厂家"=w1865, "电池类型"=w1865, "电池生产日期"=w1865) -> (w1867:T13)
                                n1148 = local write "电池信息"(w1867) -> ()
                                }
                                frame "电池包组号" {
                                n1149 = local read "电池信息"() -> (w1871:T13)
                                n1150 = Bundle By Name(cluster=w1871, "电池包组号"="") -> (w1870:T13)
                                n1151 = local write "电池信息"(w1870) -> ()
                                }
                                frame "充放电安时" {
                                w1872 = 0.0 ("累计充电总安时")
                                n1152 = local read "电池信息"() -> (w1874:T13)
                                n1153 = Bundle By Name(cluster=w1874, "累计充电总安时"=w1872, "累计放电总安时"=w1872) -> (w1873:T13)
                                n1154 = local write "电池信息"(w1873) -> ()
                                }
                                frame "电池充放电次数" {
                                w1875 = 0.0 ("累计充电总安时")
                                n1155 = local read "电池信息"() -> (w1877:T13)
                                n1156 = Bundle By Name(cluster=w1877, "电池充满次数"=w1875, "电池放空次数"=w1875, "电池充电次数"=w1875) -> (w1876:T13)
                                n1157 = local write "电池信息"(w1876) -> ()
                                }
                                }
                              }
                              frame "从板" {
                                n1158 = case shown="\"电压起始值\"" w1878 {
                                frame "假", Default {
                                }
                                frame "电压起始值" {
                                n1159 = control-ref of="项目信息 2"() -> (w1879:refnum<vi>)
                                n1160 = for {
                                N: 1 -> [_]
                                tunnel: [""] -> w1883 mode=indexing
                                }
                                n1161 = call "表格数据输入-8.6.vi"("行数"=u32 0, "列数"=u32 1, "字符串数组"=w1883, "表格引用"=w1879) -> ()  [unwired: 8 in]
                                }
                                frame "通道电压个数" {
                                n1162 = control-ref of="项目信息 2"() -> (w1885:refnum<vi>)
                                n1163 = for {
                                N: 5 -> [_]
                                tunnel: [""] -> w1889 mode=indexing
                                }
                                n1164 = call "表格数据输入-8.6.vi"("行数"=u32 22, "列数"=u32 1, "字符串数组"=w1889, "表格引用"=w1885) -> ()  [unwired: 8 in]
                                }
                                frame "保险位置" {
                                n1165 = control-ref of="项目信息 2"() -> (w1891:refnum<vi>)
                                n1166 = for {
                                N: 10 -> [_]
                                tunnel: [""] -> w1895 mode=indexing
                                }
                                n1167 = call "表格数据输入-8.6.vi"("行数"=u32 2, "列数"=u32 1, "字符串数组"=w1895, "表格引用"=w1891) -> ()  [unwired: 8 in]
                                }
                                frame "温度起始值" {
                                n1168 = control-ref of="项目信息 2"() -> (w1897:refnum<vi>)
                                n1169 = for {
                                N: 1 -> [_]
                                tunnel: [""] -> w1901 mode=indexing
                                }
                                n1170 = call "表格数据输入-8.6.vi"("行数"=u32 1, "列数"=u32 1, "字符串数组"=w1901, "表格引用"=w1897) -> ()  [unwired: 8 in]
                                }
                                frame "加热控制参数" {
                                n1171 = local write "加热控制参数"(T11 {"风机开启温度"=0.0, "风机关闭温度"=0.0, "加热开启温度"=0.0, "加热关闭温度"=0.0, "风机开启温差"=0.0, "风机关闭温差"=0.0, "加热关闭温差"=0.0} ("加热控制参数")) -> ()
                                }
                                frame "一级故障阀值" {
                                n1172 = local write "一级故障 6"(T15 {"电压过高"=0.0, "电压过低"=0.0, "温度过高"=0.0, "温度过低"=0.0, "电压不均衡(V)"=0.0, "温度不均衡"=0.0, "SOC过低"=0.0} ("一级故障 6")) -> ()
                                }
                                frame "二级故障阀值" {
                                n1173 = local write "一级故障 7"(T15 {"电压过高"=0.0, "电压过低"=0.0, "温度过高"=0.0, "温度过低"=0.0, "电压不均衡(V)"=0.0, "温度不均衡"=0.0, "SOC过低"=0.0} ("一级故障 7")) -> ()
                                }
                                frame "三级故障阀值" {
                                n1174 = local write "一级故障 8"(T15 {"电压过高"=0.0, "电压过低"=0.0, "温度过高"=0.0, "温度过低"=0.0, "电压不均衡(V)"=0.0, "温度不均衡"=0.0, "SOC过低"=0.0} ("一级故障 7")) -> ()
                                }
                                frame "均衡参数" {
                                n1175 = local write "均衡参数"(T17 {"充电结束电压(90%)"=0.0, "充电结束电压(91%)"=0.0, "充电结束电压(92%)"=0.0, "充电结束电压(93%)"=0.0, "充电结束电压(94%)"=0.0, "均衡计算-电压高阀值1级"=0.0, "均衡计算-电压高阀值2级"=0.0, "均衡计算-电压低阀值1级"=0.0, "均衡计算-电压低阀值2级"=0.0, "均衡计算-最低电压阀值"=0.0, "均衡停止-最低电压阀值"=0.0, "均衡计算-电压极差阀值"=0.0, "充电结束电压(95%)"=0.0, "充电结束电压(96%)"=0.0, "充电结束电压(97%)"=0.0, "充电结束电压(98%)"=0.0, "充电结束电压(99%)"=0.0, "充电结束电压(100%)"=0.0} ("均衡参数")) -> ()
                                }
                                frame "均衡阀值" {
                                w1908 = sgl 0.0 ("均衡计算-电压高阀值1级")
                                n1176 = local read "均衡参数"() -> (w1909:T17)
                                n1177 = Bundle By Name(cluster=w1909, "均衡计算-电压高阀值1级"=w1908, "均衡计算-电压高阀值2级"=w1908, "均衡计算-电压低阀值1级"=w1908, "均衡计算-电压低阀值2级"=w1908, "均衡计算-最低电压阀值"=w1908, "均衡停止-最低电压阀值"=w1908, "均衡计算-电压极差阀值"=w1908) -> (w1910:T17)
                                n1178 = local write "均衡参数"(w1910) -> ()
                                }
                                frame "充电结束电压" {
                                w1911 = sgl 0.0 ("均衡计算-电压高阀值1级")
                                n1179 = local read "均衡参数"() -> (w1912:T17)
                                n1180 = Bundle By Name(cluster=w1912, "充电结束电压(90%)"=w1911, "充电结束电压(91%)"=w1911, "充电结束电压(92%)"=w1911, "充电结束电压(93%)"=w1911, "充电结束电压(94%)"=w1911, "充电结束电压(95%)"=w1911, "充电结束电压(96%)"=w1911, "充电结束电压(97%)"=w1911, "充电结束电压(98%)"=w1911, "充电结束电压(99%)"=w1911, "充电结束电压(100%)"=w1911) -> (w1913:T17)
                                n1181 = local write "均衡参数"(w1913) -> ()
                                }
                                }
                              }
                            }
                          }
                          frame #1 {
                            w1914 = FALSE ("流控帧")
                            w1915 = TRUE ("流控帧 2")
                            n1182 = global write "EV05全局变量1.vi" "写入超时"(w1914) -> ()
                            n1183 = global write "EV05全局变量1.vi" "流控帧"(w1914) -> ()
                            n1184 = local write "写?"(w1914) -> ()
                            n1185 = local write "消除"(w1915) -> ()
                            n1186 = local write "控制1"(w1915) -> ()
                            n1187 = global write "EV05全局变量1.vi" "流控帧 2"(w1915) -> ()
                            n1188 = local write "写入超时"(w1914) -> ()
                            "流控帧" <- w1914
                            "流控帧 2" <- w1915
                          }
                          frame #2 {
                            n1189 = Wait Until Next ms Multiple(millisecond multiple=u32 300 ("毫秒倍数")) -> ()  [unwired: 1 out]
                          }
                          frame #3 {
                            n1190 = local read "设备索引号"() -> (w1918:u16)
                            n1191 = local read "CAN卡类型"() -> (w1919:u32)
